vi "CLD 1 Elapsed Time Express Self Solution.vi"() -> ()   [LabVIEW 2015]
doc: "LabVIEW CLD 1 Exercise"
panel:
  out "error out":errorcluster
  in  "error in":errorcluster
  out "Elapsed Time":string
  out "Time has Elapsed":bool
  in  "Auto Reset":bool=TRUE
  in  "Reset Button":bool
  in  "Stop VI":bool
  in  "Time Target (s)":dbl=2.0
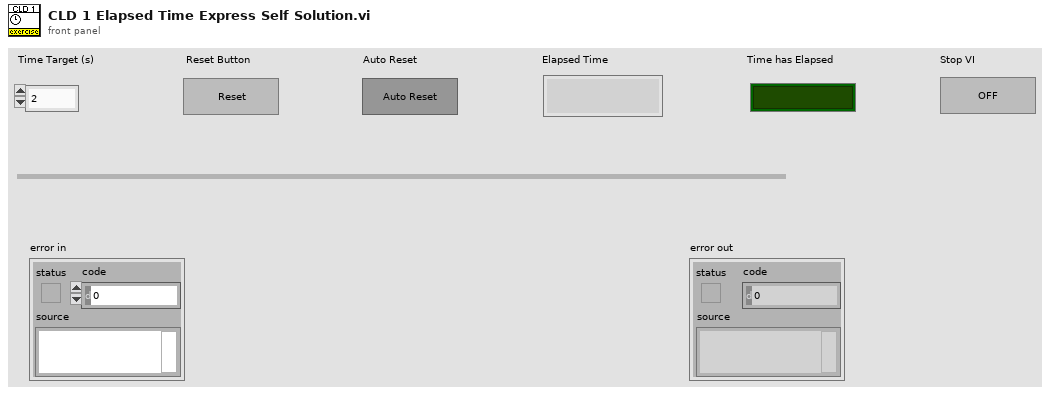
[diagram p1: front panel]
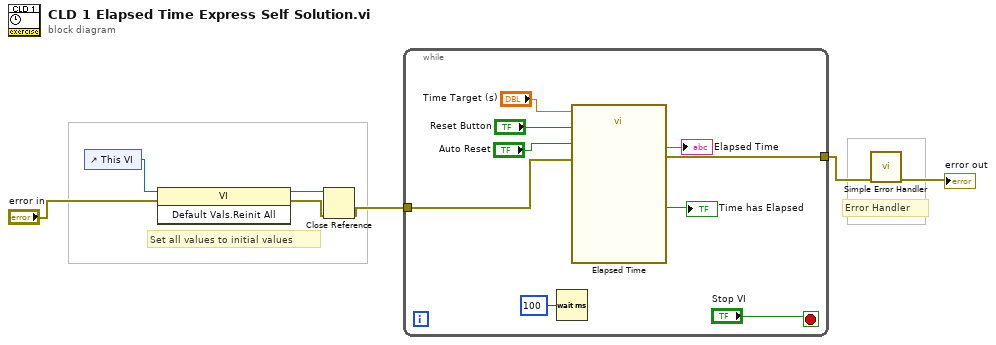
[diagram p0: block diagram]
diagram:
  # "Error Handler"
  # "Set all values to initial values"
  n1 = control-ref of="This VI"() -> (w7:refnum<vi>)
  n2 = invoke class="VI" method="Default Vals.Reinit All"(reference=w7, error in="error in") -> (reference out=w5:refnum<vi>, error out=w4:errorcluster)  [unwired: 1 in, 1 out]
  n3 = Close Reference(reference=w5, error in (no error)=w4) -> (error out=w3:errorcluster)
  n4 = while {
    tunnel: w3 -> [w13]
    tunnel: [w10] -> w2
    stop <- "Stop VI" stop-if-true
    n5 = Wait (ms)(milliseconds to wait=u32 100) -> ()  [unwired: 1 out]
    n6 = call "Elapsed Time"("Time Target (s)"="Time Target (s)", "Reset"="Reset Button", "Auto Reset"="Auto Reset", "error in (no error)"=w13) -> ("Time has Elapsed"=→"Time has Elapsed":bool, "Elapsed Time Text"=→"Elapsed Time":string, "error out"=w10:errorcluster)  [unwired: 8 in, 5 out]
  }
  n7 = call <vilib>:"Simple Error Handler.vi"("error in (no error)"=w2) -> ("error out"=→"error out":errorcluster)  [unwired: 4 in, 4 out]
